vi "Send Write Mode.vi"(7 "Message Priority (Normal)":T2=enum."Normal", 8 "error in (no error)":errorcluster, 10 "Mode":T1, 11 "Message Enqueuer":refnum<class "Message Enqueuer.lvclass">) -> (0 "error out":errorcluster, 3 "Message Enqueuer out":refnum<class "Message Enqueuer.lvclass">)   [LabVIEW 2019, in "Multimeter.lvlib" / "Write Mode Msg.lvclass"]
doc: "This VI sends the message to an actor."
uses:
  Write Mode Msg.lvclass
  builds/Engine/Actor Framework.lvlibp/1abvi3w/vi.lib/ActorFramework/Message Enqueuer/Message Enqueuer.lvclass
  builds/Engine/Actor Framework.lvlibp/1abvi3w/vi.lib/ActorFramework/Message Enqueuer/Message Priority.ctl
  Custom Controls/Mode.ctl
  Write Mode Msg.lvclass/Write Mode Msg.ctl
  C:/Users/Public/Documents/Development/builds/Engine/Actor Framework.lvlibp/1abvi3w/vi.lib/ActorFramework/Message/Message.lvclass
  Library/Multimeter.lvclass
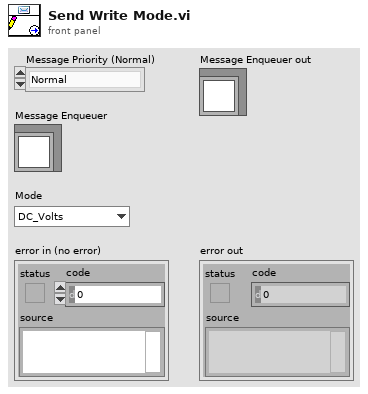
[diagram p1: front panel]
types:
  T1 = typedef "Multimeter.lvlib/Multimeter.lvclass/Mode.ctl" = enum16{"DC_Volts", "AC_Volts", "DC_Current", "AC_Current", "Resistance_2_Wire", "Resistance_4_Wire", "Diode", "Frequency", "Period", "AC_Volts_DC_Coupled", "Capacitance", "Inductance", "Temperature"}
  T2 = typedef "Actor Framework.lvlibp/Message Enqueuer.lvclass/Message Priority.ctl" = enum16{"Low", "Normal", "High"}
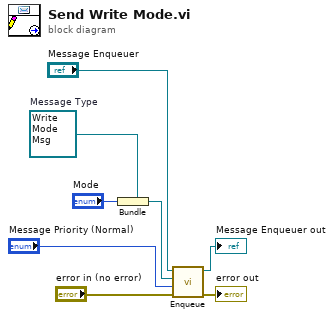
[diagram p0: block diagram]
diagram:
  w5 = refnum<class "Write Mode Msg.lvclass"> refnum  # Message Type
  n1 = Bundle(cluster=w5, "Mode") -> (w4:refnum<class "Write Mode Msg.lvclass">)
  n2 = call "Enqueue.vi"("error in (no error)"="error in (no error)", "Message Priority (Normal)"="Message Priority (Normal)", "Message"=w4, "Message Enqueuer in"="Message Enqueuer") -> ("error out"=→"error out":errorcluster, "Message Enqueuer out"=→"Message Enqueuer out":refnum<class "Message Enqueuer.lvclass">)  [unwired: 6 in]
